vi "Configure Percent.vi"(0 "VISA resource name":refnum<visa-resource-name>, 5 "error in (no error)":errorcluster, 6 "State":bool, 9 "Target Value":dbl) -> (14 "VISA resource name out":refnum<visa-resource-name>, 19 "error out":errorcluster)   [LabVIEW 2020, in "Keithley 2100 Series.lvlib"]
doc: "Definition:\nThis mathematical function calculates the ratio of a measurement reading to a specified target value as the form of percentage.\n\nThe specified target value is store in a volatile memory and will be cleared after the meter has been turned off or a remote interface reset.\n\nRemote Interface Operation:\nUse the following commands to enable and configure Percent function:\n\nCALCulate:FUNCtion PERCent\nCALCulate:STATe {OFF|ON}\nCALCulate:STATe?\nCALCulate:PERCent:TARGet {<value>|MINimum|MAXimum}\nCALCulate:PERCent:TARGet? [MINimum|MAXimum]"
uses:
  Keithley 2100 Series.lvlib
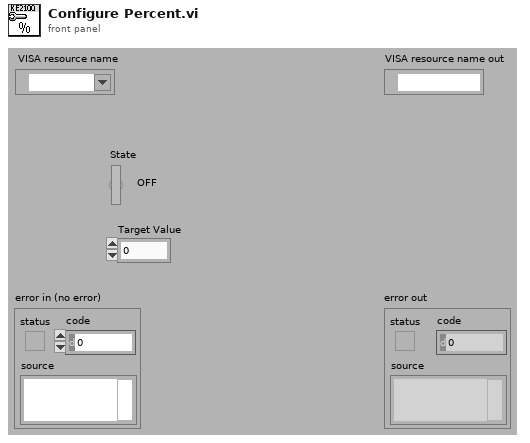
[diagram p1: front panel]
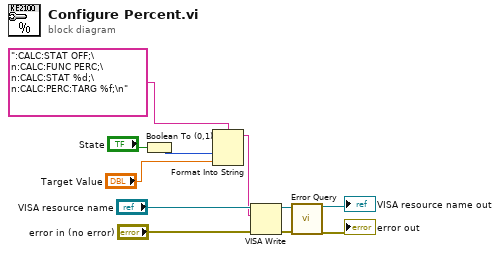
[diagram p0: block diagram]
diagram:
  n1 = Boolean To (0,1)(Boolean="State") -> (0, 1=w4:i16)
  n2 = Format Into String(format string=":CALC:STAT OFF;\n:CALC:FUNC PERC;\n:CALC:STAT %d;\n:CALC:PERC:TARG %f;\n", w4, "Target Value") -> (resulting string=w5:string)  [unwired: 2 in, 1 out]
  n3 = VISA Write(VISA resource name="VISA resource name", write buffer=w5, error in (no error)="error in (no error)") -> (VISA resource name out=w10:refnum<visa-resource-name>, error out=w11:errorcluster)  [unwired: 1 out]
  n4 = call "Error Query.vi"("VISA resource name"=w10, "error in (no error)"=w11) -> ("VISA resource name out"=→"VISA resource name out":refnum<visa-resource-name>, "error out"=→"error out":errorcluster)  [unwired: 14 in, 2 out]
